vi "NI VeriStand - Get Loop Type.vi"(8 "error in (no error)":errorcluster, 11 "Device Ref in":T2 format="%.0x") -> (0 "error out":errorcluster, 1 "Use Device Clock":bool, 2 "Loop type":T1, 3 "Device Ref out":T2 format="%.0x")   [LabVIEW 2020, in "Custom Device API.lvlib"]
doc: "Returns the type of loop (While Loop or Timed Loop) that an asynchronous custom device uses. If <B>Loop type</B> is 1 - Timed Loop, this VI also returns whether the loop uses the device clock as its timing source."
uses:
  <vilib>/NI VeriStand/Custom Device API/Custom Device API.lvlib
  <vilib>/NI VeriStand/Custom Device API/Custom Device Item Ref.ctl
  <vilib>/NI VeriStand/Custom Device API/Custom Device Loop Type.ctl
  d67e76c5-2ea8-40ec-a208-052e07854456.vi
  <vilib>/NI VeriStand/Custom Device API/Custom Device Offline Path.vi
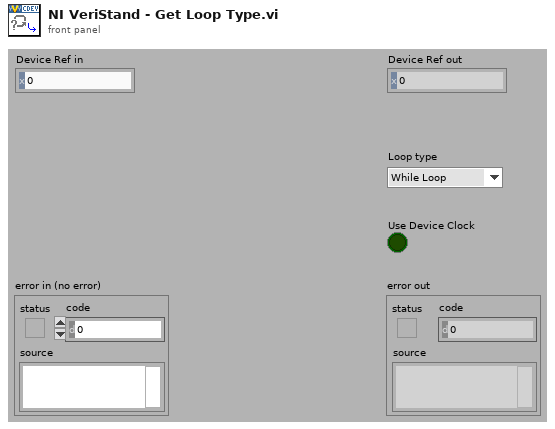
[diagram p1: front panel]
types:
  T1 = typedef "Custom Device API.lvlib/Custom Device Loop Type.ctl" = enum32{"While Loop", "Timed Loop"}
  T2 = typedef "Custom Device API.lvlib/Custom Device Item Ref.ctl" = u64
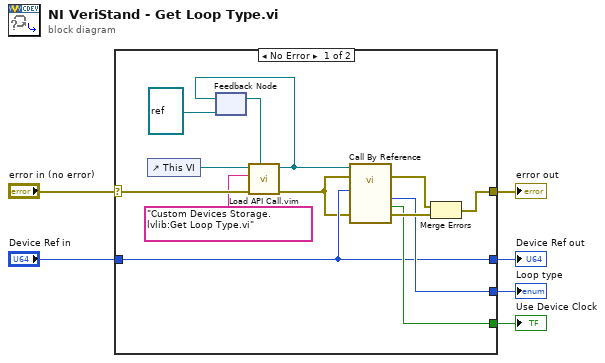
[diagram p0: block diagram]
diagram:
  n1 = case shown="No Error" "error in (no error)" {
    selector: "error in (no error)" -> [w12 w21]
    tunnel: [w18 w21] -> w6
    tunnel: "Device Ref in" -> [w15 w20]
    tunnel: [w15 w20] -> w4
    tunnel: [w17 _] -> w3
    tunnel: [w16 _] -> w2
    frame No Error {
      n2 = control-ref of="This VI"() -> (w13:refnum<vi>)
      n3 = feedback #1(refnum<vi> refnum ("type specifier VI Refnum (for type only)")) -> (w14:refnum<vi>)
      n4 = call "Load API Call.vim"("VI reference in"=w14, "error in (no error)"=w12, "VI qualified name"="Custom Devices Storage.lvlib:Get Loop Type.vi", "Caller VI ref"=w13) -> ("error out"=w11:errorcluster, "VI reference"=w10:refnum<vi>)  [unwired: 6 in]
      n5 = feedback-in #1(w10) -> ()
      n6 = call-by-ref "?"(reference=w10, error in=w11, 8:"error in (no error)"=w11, "Device Ref in"=w15) -> (error out=w7:errorcluster, 0:"error out"=w19:errorcluster, "Use Device Clock"=w16:bool, "Loop type"=w17:T1)  [unwired: 6 in, 2 out]
      n7 = Merge Errors(w7, w19) -> (w18:errorcluster)
    }
    frame Error {
    }
  }
  "Device Ref out" <- w4
  "error out" <- w6
  "Loop type" <- w3
  "Use Device Clock" <- w2
